vi "Power Accuracy System Warning.vi"(6 "Driver Ref (null)":T9, 7 "Coerced PV Test Parameters":T1={"Stimulus"={"Power Start"=38, "Power Stop"=46, "Frequency Type"=enum."Band Edges", "Frequency Points"=[], "TX 1 Frequency (MHz)"={"Min"=0.0, "Max"=0.0}, "TX 2 Frequency (MHz)"={"Min"=0.0, "Max"=0.0}, "RX Frequency (MHz)"={"Min"=0.0, "Max"=0.0}, "Pad Model Number"="", "Pad Serial Number"="", "Pad Values"=[]}, "Measurement"={"DUT Port"=enum."Port 1", "Direction"=0}, "Display"={"Power"={"Min"=0, "Max"=0}, "Tolerance"={"Min"=0.0, "Max"=0.0}}, "Limit"={"Tolerance"=0.35}, "Calibration"={"Calibrated?"=FALSE}} {"Measurement"."Direction" items=["Reverse", "Forward", "Auxiliary"]}, 10 "PV Test Parameters":T1={"Stimulus"={"Power Start"=38, "Power Stop"=46, "Frequency Type"=enum."Band Edges", "Frequency Points"=[], "TX 1 Frequency (MHz)"={"Min"=0.0, "Max"=0.0}, "TX 2 Frequency (MHz)"={"Min"=0.0, "Max"=0.0}, "RX Frequency (MHz)"={"Min"=0.0, "Max"=0.0}, "Pad Model Number"="", "Pad Serial Number"="", "Pad Values"=[]}, "Measurement"={"DUT Port"=enum."Port 1", "Direction"=0}, "Display"={"Power"={"Min"=0, "Max"=0}, "Tolerance"={"Min"=0.0, "Max"=0.0}}, "Limit"={"Tolerance"=0.35}, "Calibration"={"Calibrated?"=FALSE}} {"Measurement"."Direction" items=["Reverse", "Forward", "Auxiliary"]}, 11 "TestSetDef":T10={"General"={"ID"=0, "Model"="", "Dual Port?"=FALSE, "Options"="", "Options"={"E"=FALSE, "K"=FALSE, "H"=FALSE, "W"=FALSE, "F"=FALSE}, "Cal File"=path ""}, "Receiver"={"Fstart, MHz"=0.0, "Fstop MHz"=0.0, "Fstep MHz"=0.0, "IF, MHz"=0.0}, "RX Band"={"Fstart, MHz"=0.0, "Fstop MHz"=0.0}, "TX 1"={"Fstart, MHz"=0.0, "Fstop MHz"=0.0, "Pmax, dBm"=0.0, "Pstep, dB"=0.0}, "TX 2"={"Fstart, MHz"=0.0, "Fstop MHz"=0.0, "Pmax, dBm"=0.0, "Pstep, dB"=0.0}, "Low-side?"=TRUE}) -> (2 "Message (\"\")":string="\n\n", 3 "Abort?":bool)   [LabVIEW 2011]
uses:
  SI.LIB/PIM.LIB/HW IO/Test Set Definition.ctl
  TypeDefs/Power Accuracy Test Parameters.ctl
  TypeDefs/Power Accuracy Stimulus Parameters.ctl
  TypeDefs/Power Accuracy Measurement Parameters.ctl
  SI.LIB/PIM.LIB/HW IO/DUTport.ctl
  SI.LIB/PIM.LIB/HW IO/MeasMode.ctl
  TypeDefs/Power Accuracy Display Parameters.ctl
  TypeDefs/Power Accuracy Limit Parameters.ctl
  TypeDefs/Power Accuracy Calibration State.ctl
  drivers/PIM/PIM Driver Ref.ctl
  drivers/PIM/PIM Command.ctl
panel:
  in  "B 2":bool
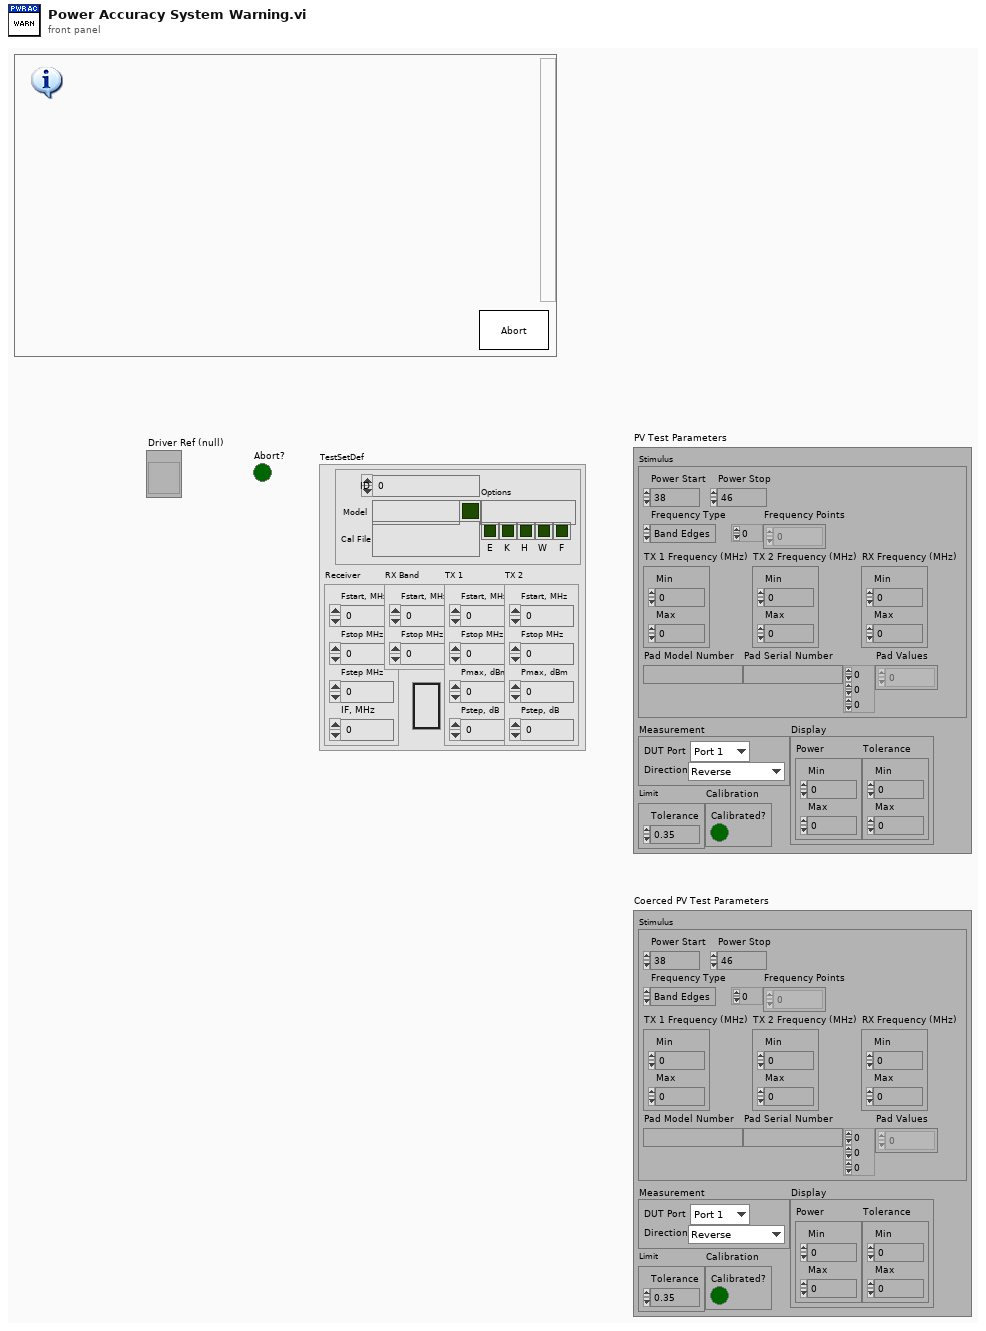
[diagram p1: front panel]
types:
  T1 = typedef "Power Accuracy Test Parameters.ctl" = cluster{"Stimulus":T2, "Measurement":T3, "Display":T6, "Limit":T7, "Calibration":T8}
  T2 = typedef "Power Accuracy Stimulus Parameters.ctl" = cluster{"Power Start":i32, "Power Stop":i32, "Frequency Type":enum16{"Band Edges", "Custom"}, "Frequency Points":dbl[], "TX 1 Frequency (MHz)":cluster{"Min":dbl, "Max":dbl}, "TX 2 Frequency (MHz)":cluster{"Min":dbl, "Max":dbl}, "RX Frequency (MHz)":cluster{"Min":dbl, "Max":dbl}, "Pad Model Number":string, "Pad Serial Number":string, "Pad Values":dbl[][][]}
  T3 = typedef "Power Accuracy Measurement Parameters.ctl" = cluster{"DUT Port":T4, "Direction":T5}
  T4 = typedef "DUTport.ctl" = enum16{"Port 1", "Port 2"}
  T5 = typedef "MeasMode.ctl" = u16
  T6 = typedef "Power Accuracy Display Parameters.ctl" = cluster{"Power":cluster{"Min":i32, "Max":i32}, "Tolerance":cluster{"Min":dbl, "Max":dbl}}
  T7 = typedef "Power Accuracy Limit Parameters.ctl" = cluster{"Tolerance":dbl}
  T8 = typedef "Power Accuracy Calibration State.ctl" = cluster{"Calibrated?":bool}
  T9 = typedef "PIM Driver Ref.ctl" = refnum<vi>
  T10 = typedef "Test Set Definition.ctl" = cluster{"General":cluster{"ID":u32, "Model":string, "Dual Port?":bool, "Options":string, "Options":cluster{"E":bool, "K":bool, "H":bool, "W":bool, "F":bool}, "Cal File":path}, "Receiver":cluster{"Fstart, MHz":dbl, "Fstop MHz":dbl, "Fstep MHz":dbl, "IF, MHz":dbl}, "RX Band":cluster{"Fstart, MHz":dbl, "Fstop MHz":dbl}, "TX 1":cluster{"Fstart, MHz":dbl, "Fstop MHz":dbl, "Pmax, dBm":dbl, "Pstep, dB":dbl}, "TX 2":cluster{"Fstart, MHz":dbl, "Fstop MHz":dbl, "Pmax, dBm":dbl, "Pstep, dB":dbl}, "Low-side?":bool}
  T11 = typedef "PIM Command.ctl" = enum16{"LOAD", "KEEP ALIVE", "VALIDATE", "INITIALIZE", "PRESET", "GET CALIBRATION", "SET STIMULUS", "TOGGLE TX POWER", "SET TX ON", "SET TX OFF", "MEASURE", "UNLOAD"}
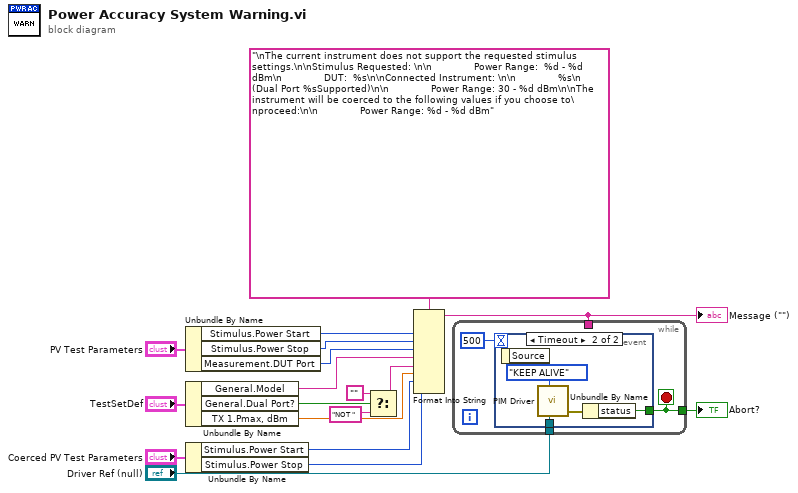
[diagram p0: block diagram]
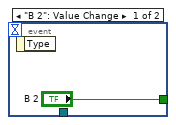
[diagram p2: hidden frame]
diagram:
  n1 = Unbundle By Name("PV Test Parameters") -> ("Stimulus.Power Start"=w8:i32, "Stimulus.Power Stop"=w7:i32, "Measurement.DUT Port"=w6:T4)
  n2 = Unbundle By Name("TestSetDef") -> ("General.Model"=w16:string, "General.Dual Port?"=w11:bool, "TX 1.Pmax, dBm"=w5:dbl)
  n3 = Unbundle By Name("Coerced PV Test Parameters") -> ("Stimulus.Power Start"=w3:i32, "Stimulus.Power Stop"=w2:i32)
  n4 = Select(t="", s=w11, f="NOT " ("string")) -> (s? t:f=w1:string)
  n5 = Format Into String(format string="\nThe current instrument does not support the requested stimulus settings.\n\nStimulus Requested: \n\n              Power Range:  %d - %d dBm\n              DUT:  %s\n\nConnected Instrument: \n\n              %s\n              (Dual Port %sSupported)\n\n              Power Range: 30 - %d dBm\n\nThe instrument will be coerced to the following values if you choose to\nproceed:\n\n              Power Range: %d - %d dBm", w8, w7, w6, w16, w1, w5, w3, w2) -> (resulting string=w10:string)  [unwired: 2 in, 1 out]
  "Message (\"\")" <- w10
  n6 = while {
    tunnel: [w21] -> w18
    tunnel: w10 -> [_]
    tunnel: "Driver Ref (null)" -> [w19]
    stop <- w21 stop-if-true
    n7 = event shown="[1] Timeout" {
      selector: _ -> [_ _]
      dyn-events: _ -> [_ _]
      timeout: 500 -> [_ _]
      tunnel: ["B 2" w24] -> w21
      tunnel: w19 -> [_ w23]
      event "B 2": Value Change {
        n8 = event-data() -> ()  [unwired: 2 out]
      }
      event Timeout {
        n9 = event-data() -> ()  [unwired: 2 out]
        n10 = call "PIM Driver.vi"("Driver Ref (null)"=w23, "PIM Command"=PIM_Command."KEEP ALIVE") -> ("error out"=w25:errorcluster)  [unwired: 3 in, 6 out]
        n11 = Unbundle By Name(w25) -> ("status"=w24:bool)
      }
    }
  }
  "Abort?" <- w18
